vi "create new channel.vi"(9 "channel classification":T1, 10 "data type":T2, 11 "channel name":string) -> (3 "channel":refnum<class "TBM channel.lvclass">)   [LabVIEW 2013, in "TBM channel.lvclass"]
doc: "Constructs a new channel using a name, type, and direction/classification. This constructor does not set any other properties of the class, but they are settable using property nodes."
uses:
  TBM channel.lvclass
  <vilib>/NI/Tag Bus/tag/Data Type.ctl
  channel classification.ctl
  TBM channel.lvclass/TBM channel.ctl
  <vilib>/NI/Tag Bus/tag/tag descriptor.lvclass/tag descriptor.ctl
  <vilib>/NI/Tag Bus/tag/tag descriptor.lvclass
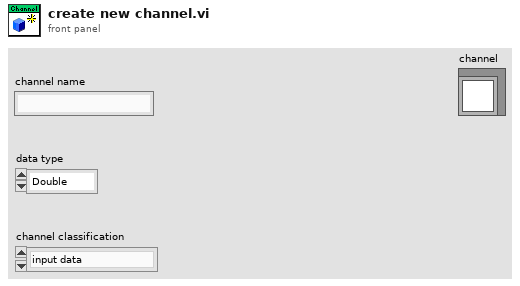
[diagram p1: front panel]
types:
  T1 = typedef "TBM channel.lvclass/channel classification.ctl" = enum16{"input data", "output data", "processing parameter", "processing result"}
  T2 = typedef "tag bus.lvlib/tag descriptor.lvclass/Data Type.ctl" = enum16{"Double", "Single", "I64", "I32", "I16", "I8", "U64", "U32", "U16", "U8", "Boolean", "String", "Array of Double", "Array of Single", "Array of I64", "Array of I32", "Array of I16", "Array of I8", "Array of U64", "Array of U32", "Array of U16", "Array of U8", "Array of Boolean", "Array of String"}
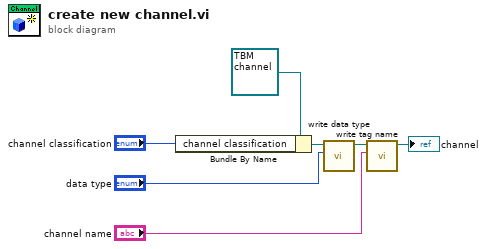
[diagram p0: block diagram]
diagram:
  n1 = Bundle By Name(cluster=refnum<class "TBM channel.lvclass"> refnum ("channel in"), "channel classification"="channel classification") -> (w6:refnum<class "TBM channel.lvclass">)
  n2 = call <vilib>:"write data type.vi"("data type"="data type", "system tag in"=w6) -> ("system tag out"=w3:refnum<class "TBM channel.lvclass">)  [unwired: 8 in, 1 out]
  n3 = call <vilib>:"write tag name.vi"("name"="channel name", "system tag in"=w3) -> ("system tag out"=→"channel":refnum<class "TBM channel.lvclass">)  [unwired: 8 in, 1 out]
